vi "Index from Control Ref.vi"(8 "error in (no error)":errorcluster, 10 "Ctl Refnum In":refnum<vi>, 11 "ControlArray in":refnum<class "ControlArray.lvclass">) -> (0 "error out":errorcluster, 1 "Index":i32, 2 "Ctl Refnum":refnum<vi>, 3 "ControlArray out":refnum<class "ControlArray.lvclass">)   [LabVIEW 2020, in "Control Array.lvlib" / "ControlArray.lvclass"]
doc: "Determines the current array position represented by a control reference. This is generated based on which index within the controls the reference is as well as the current scroll position. A value of -1 means the reference currently does not map to a value, for instance if the array is too small to utilize the specified control."
uses:
  ControlArray.lvclass
  ControlArray.lvclass/ControlArray.ctl
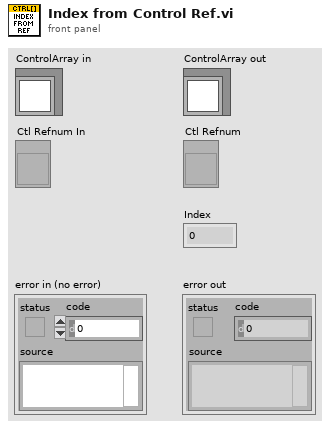
[diagram p1: front panel]
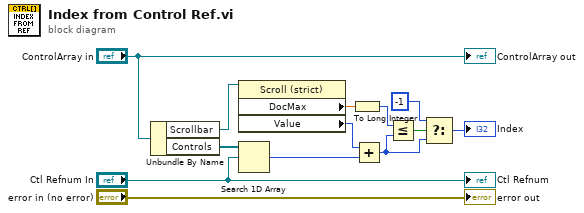
[diagram p0: block diagram]
diagram:
  n1 = Unbundle By Name("ControlArray in") -> ("Scrollbar"=w9:refnum<vi>, "Controls"=w11:refnum<vi>[])
  n2 = property class="Scroll (strict)"(reference=w9) -> ("DocMax"=w6:dbl, "Value"=w7:i32)  [unwired: 1 in, 2 out]
  n3 = Search 1D Array(1D array=w11, element="Ctl Refnum In") -> (index of element=w8:i32)  [unwired: 1 in]
  n4 = To Long Integer(number=w6) -> (32bit integer=w5:i32)
  n5 = Add(x=w7, y=w8) -> (x+y=w3:i32)
  n6 = Less Or Equal?(x=w5, y=w3) -> (x <= y?=w4:bool)
  n7 = Select(t=-1, s=w4, f=w3) -> (s? t:f=→"Index":i32)
  "error out" <- "error in (no error)"
  "ControlArray out" <- "ControlArray in"
  "Ctl Refnum" <- "Ctl Refnum In"
